vi "Global.vi"() -> ()   [LabVIEW 2017, in "nifxpmath_PolarToRect.xnode"]
uses:
  <vilib>/rvi/FXPMathLib/FxpPolarToRect/XNode/nifxpmath_PolarToRect.xnode
panel:
  in  "TERM PH NAME w/o UNIT":string="phase"
  out "SMALL ICON w/ 4WIRE":picture
  in  "TERM Y NAME":string="y"
  in  "TERM PH NAME":string="phase (pi)"
  in  "TERM X NAME":string="x"
  in  "TERM MA NAME":string="magnitude"
  out "SMALL ICON":picture
  out "NORMAL BANNER":picture
  in  "TERM MA ID":string="TERM_MA"
  in  "TERM Y ID":string="TERM_Y"
  in  "TERM X ID":string="TERM_X"
  in  "TERM PH ID":string="TERM_PH"
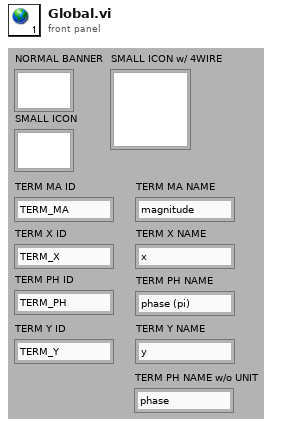
[diagram p1: front panel]
diagram:
